vi "StartSequence.vi"(8 "error in (no error)":errorcluster, 11 "Config In":T1 {"Hardware Configuration"."Lasers Configuration"."SettingValues"."785 Power" format="%.1f"; "Hardware Configuration"."Lasers Configuration"."SettingValues"."647 Power" format="%.1f"; "Hardware Configuration"."Lasers Configuration"."SettingValues"."561 Power" format="%.1f"; "Hardware Configuration"."Lasers Configuration"."SettingValues"."532 Power" format="%.1f"; "Hardware Configuration"."Lasers Configuration"."SettingValues"."488 Power" format="%.1f"; "Hardware Configuration"."Lasers Configuration"."SettingValues"."405 Power" format="%.1f"}) -> (0 "error out":errorcluster, 3 "Config Out":T1 {"Hardware Configuration"."Lasers Configuration"."SettingValues"."785 Power" format="%.1f"; "Hardware Configuration"."Lasers Configuration"."SettingValues"."647 Power" format="%.1f"; "Hardware Configuration"."Lasers Configuration"."SettingValues"."561 Power" format="%.1f"; "Hardware Configuration"."Lasers Configuration"."SettingValues"."532 Power" format="%.1f"; "Hardware Configuration"."Lasers Configuration"."SettingValues"."488 Power" format="%.1f"; "Hardware Configuration"."Lasers Configuration"."SettingValues"."405 Power" format="%.1f"})   [LabVIEW 2019]
uses:
  Settings/Settings.ctl
  Support/Hardware Configuration.ctl
  Support/Camera Configuration.ctl
  D:/SDK/PMQI-LabViewSamples/Examples/Dependencies/PVCamNET.dll
  <vilib>/vision/Image Controls.llb/IMAQ Image.ctl
  <vilib>/userdefined/High Color/IMAQdx.ctl
  E:/DevHardSoftware/MMicroscopy/HardwareAdapter/Lasers/Dependencies/Oxxius_Boxx.dll
  Lasers/Dependencies/Oxxius_Boxx.dll
  Logging/Logging Configuration.ctl
  controls/UI Configuration.ctl
  controls/CallBack Refs.ctl
  Logging/Logging.lvlib
  Settings/Settings.lvlib
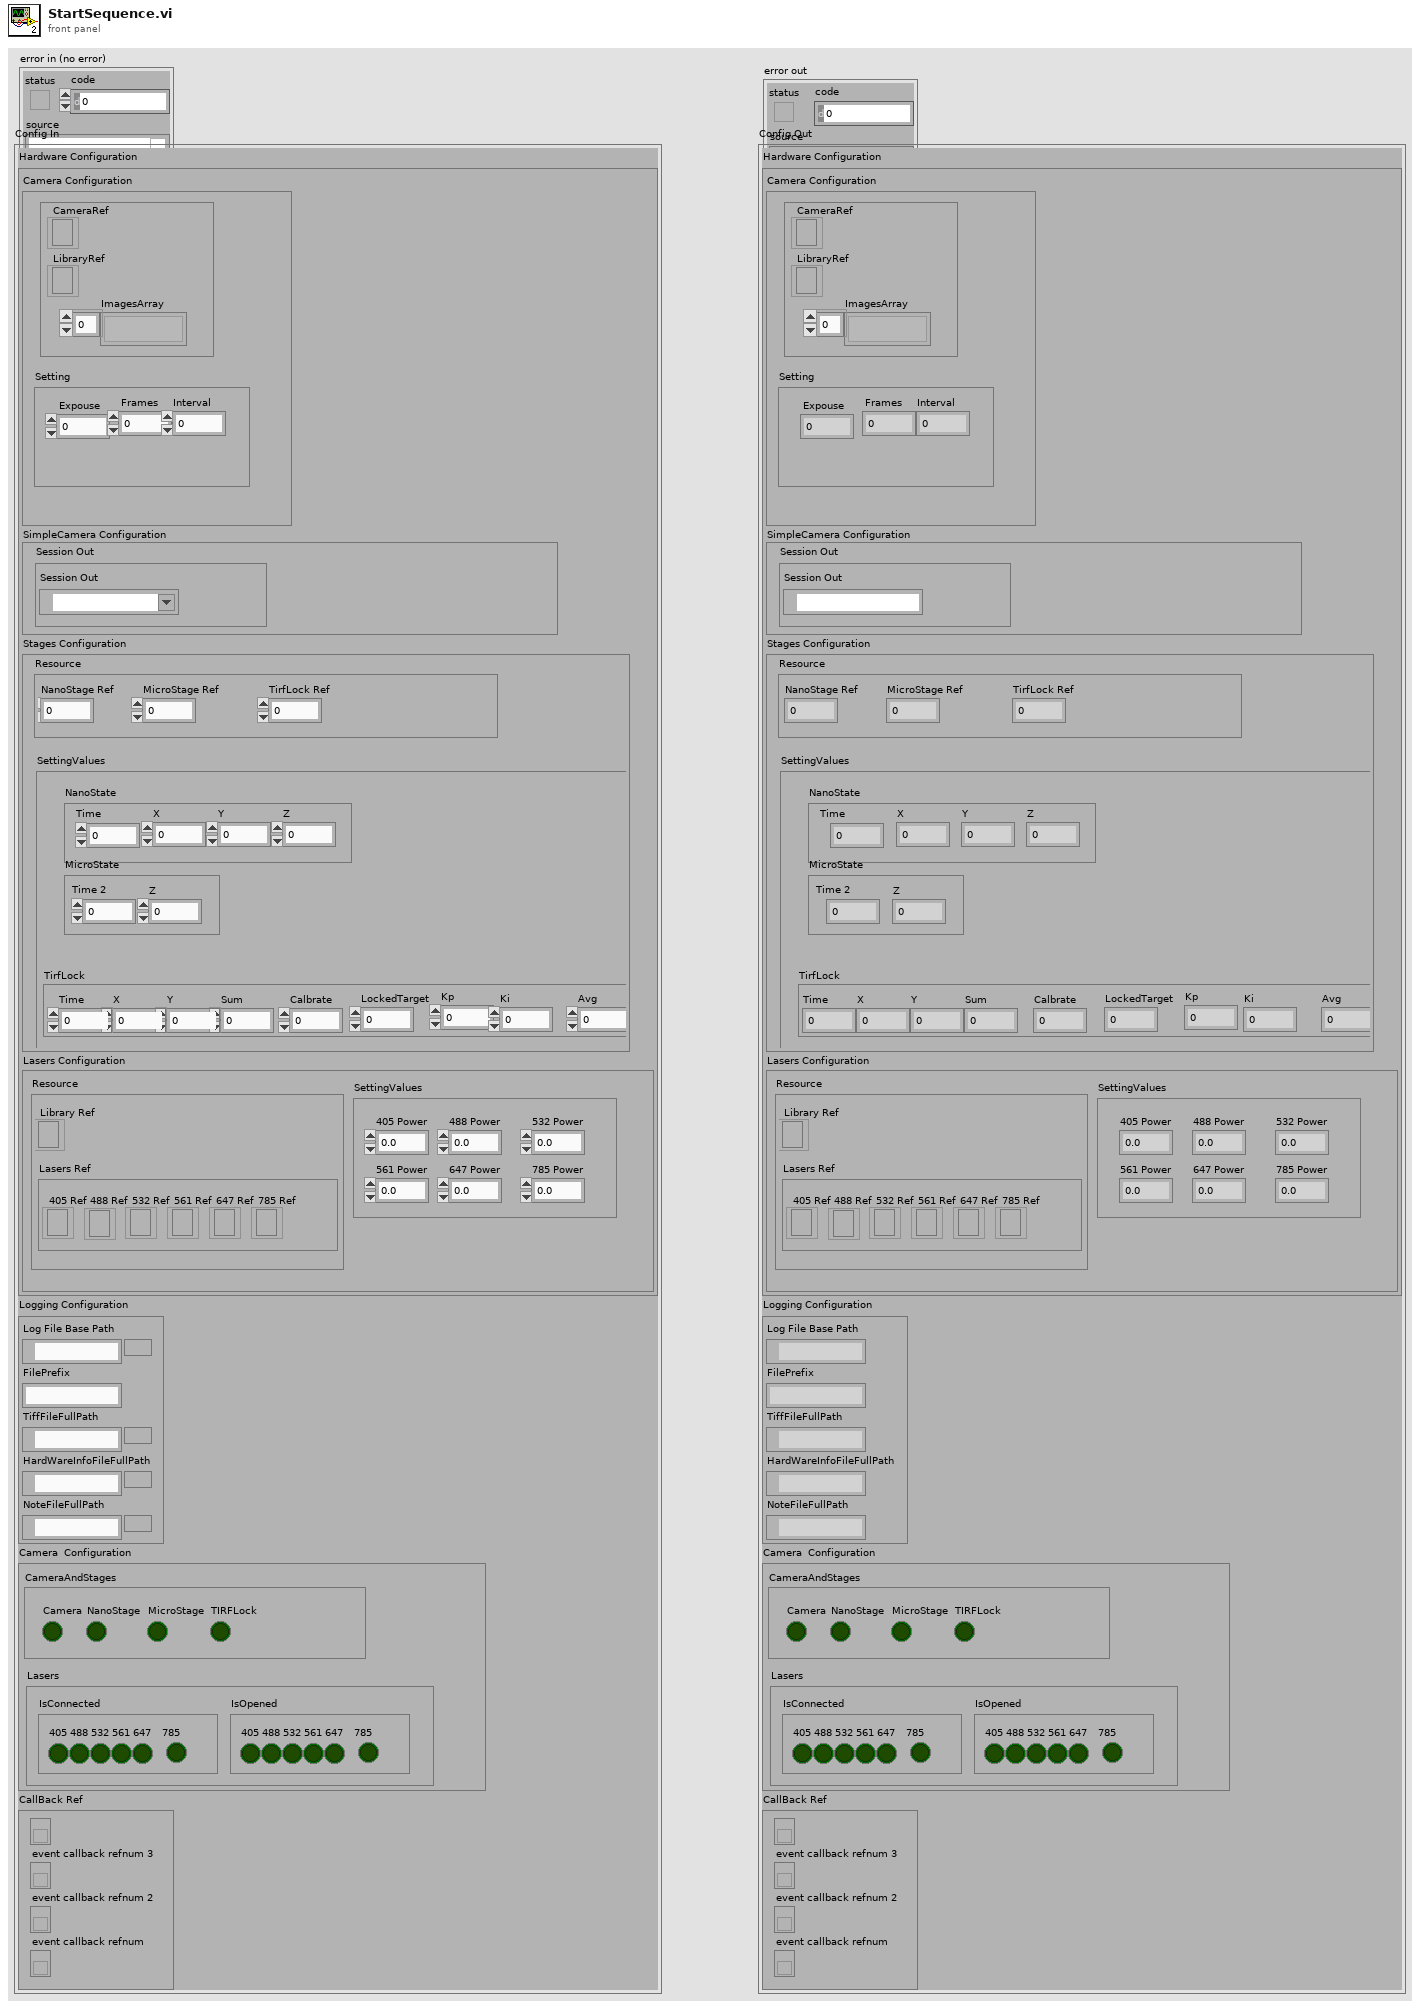
[diagram p1: front panel]
types:
  T1 = typedef "Settings.lvlib/Settings.ctl" = cluster{"Hardware Configuration":T2, "Logging Configuration":T6, "HardWare Status":cluster{"CameraAndStages":T7, "Lasers":cluster{"IsConnected":cluster{"405":bool, "488":bool, "532":bool, "561":bool, "647":bool, "785":bool}, "IsOpened":cluster{"405":bool, "488":bool, "532":bool, "561":bool, "647":bool, "785":bool}}}, "CallBack Ref":T8}
  T2 = typedef "Hardware Configuration.ctl" = cluster{"Camera Configuration":T3, "SimpleCamera Configuration":cluster{"Resource":cluster{"Session Out":T5}}, "Stages Configuration":cluster{"Resource":cluster{"NanoStage Ref":i32, "MicroStage Ref":i32, "TirfLock Ref":i32}, "SettingValues":cluster{"NanoState":cluster{"Time":dbl, "X":dbl, "Y":dbl, "Z":dbl}, "MicroState":cluster{"Time 2":dbl, "Z":dbl}, "TirfLock":cluster{"Time":dbl, "X":dbl, "Y":dbl, "Sum":dbl, "Calbrate":dbl, "LockedTarget":dbl, "Kp":dbl, "Ki":dbl, "Avg":dbl}}}, "Lasers Configuration":cluster{"SettingValues":cluster{"405 Power":sgl, "488 Power":sgl, "532 Power":sgl, "561 Power":sgl, "647 Power":sgl, "785 Power":sgl}, "Resource":cluster{"Library Ref":refnum<k24>, "Lasers Ref":cluster{"405 Ref":refnum<k24>, "488 Ref":refnum<k24>, "532 Ref":refnum<k24>, "561 Ref":refnum<k24>, "647 Ref":refnum<k24>, "785 Ref":refnum<k24>}}}}
  T3 = typedef "Camera Configuration.ctl" = cluster{"Setting":cluster{"Expouse":dbl, "Frames":dbl, "Interval":dbl}, "Resource":cluster{"CameraRef":refnum<k24>, "LibraryRef":refnum<k24>, "ImagesArray":T4[]}}
  T4 = typedef "IMAQ Image.ctl" = refnum<image>
  T5 = typedef "IMAQdx.ctl" = refnum<k21>
  T6 = typedef "Logging.lvlib/Logging Configuration.ctl" = cluster{"Log File Base Path":path, "FilePrefix":string, "TiffFileFullPath":path, "HardWareInfoFileFullPath":path, "NoteFileFullPath":path}
  T7 = typedef "UI Configuration.ctl" = cluster{"Camera":bool, "NanoStage":bool, "MicroStage":bool, "TIRFLock":bool}
  T8 = typedef "CallBack Refs.ctl" = cluster{"event callback refnum":refnum<k27>, "event callback refnum 2":refnum<k27>, "event callback refnum 3":refnum<k27>, "event callback refnum 4":refnum<k27>}
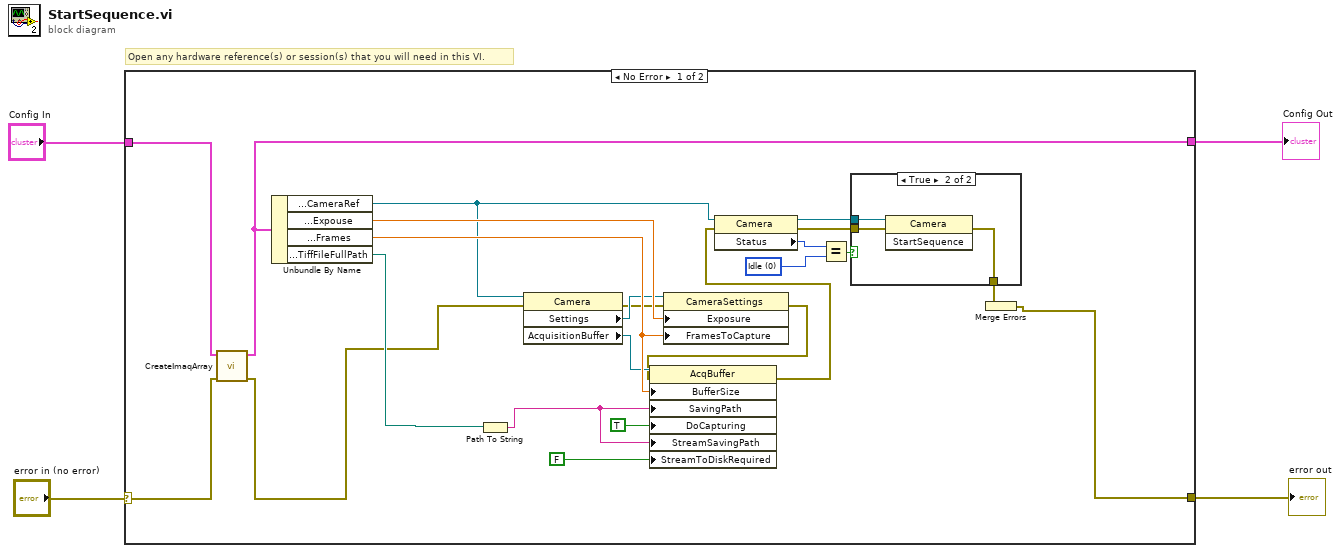
[diagram p0: block diagram]
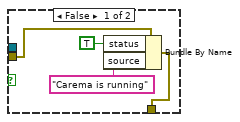
[diagram p2: hidden frame]
diagram:
  # "Open any hardware reference(s) or session(s) that you will need in this VI."
  n1 = case shown="No Error" "error in (no error)" {
    selector: "error in (no error)" -> [w7 w35]
    tunnel: [w27 w35] -> w3
    tunnel: "Config In" -> [w6 w36]
    tunnel: [w5 w36] -> w1
    frame No Error {
      w18 = 0 items=["Idle", "Capturing"] ("Status")
      n2 = call "CreateImaqArray.vi"("error in (no error)"=w7, "Config"=w6) -> ("error in (no error) 2"=w8:errorcluster, "Config 2"=w5:T1)  [unwired: 8 in]
      n3 = Unbundle By Name(w5) -> ("Hardware Configuration.Camera Configuration.Resource.CameraRef"=w24:refnum<k24>, "Hardware Configuration.Camera Configuration.Setting.Expouse"=w26:dbl, "Hardware Configuration.Camera Configuration.Setting.Frames"=w25:dbl, "Logging Configuration.TiffFileFullPath"=w23:path)
      n4 = Path To String(path=w23) -> (string=w10:string)
      n5 = property class="Camera"(reference=w24, error in=w8) -> (error out=w21:errorcluster, "Settings"=w22:refnum<k24>, "AcquisitionBuffer"=w20:refnum<k24>)  [unwired: 1 out]
      n6 = property class="CameraSettings"(reference=w22, error in=w21, "Exposure"=w26, "FramesToCapture"=w25) -> (error out=w13:errorcluster)  [unwired: 1 out]
      n7 = property class="AcqBuffer"(reference=w20, error in=w13, "BufferSize"=w25, "SavingPath"=w10, "DoCapturing"=TRUE, "StreamSavingPath"=w10, "StreamToDiskRequired"=FALSE) -> (error out=w12:errorcluster)  [unwired: 1 out]
      n8 = property class="Camera"(reference=w24, error in=w12) -> (reference out=w15:refnum<k24>, error out=w14:errorcluster, "Status"=w17:i32)
      n9 = Equal?(x=w17, y=w18) -> (x = y?=w16:bool)
      n10 = case shown="True" w16 {
        tunnel: [w28 w34] -> w19
        tunnel: w15 -> [_ w33]
        tunnel: w14 -> [w29 w32]
        frame False {
          n11 = Bundle By Name(cluster=w29, "status"=TRUE, "source"="Carema is running") -> (w28:errorcluster)
        }
        frame True {
          n12 = invoke class="Camera" method="StartSequence"(reference=w33, error in=w32) -> (error out=w34:errorcluster)  [unwired: 1 in, 2 out]
        }
      }
      n13 = Merge Errors(w19) -> (w27:errorcluster)
    }
    frame Error {
    }
  }
  "error out" <- w3
  "Config Out" <- w1
